vi "Fit Model to Plot Wrapper.vi"(0 "Fit Plot Info":T1, 11 "error in (no error)":errorcluster) -> (1 "Fitted Plot":cluster{"X Array":dbl[], "Y Array":dbl[]}, 2 "Graph Name":string, 3 "Plot Name":string, 4 "Best Fit":dbl[](array[numeric]), 6 "Fit Parameter Names":string[](array[string]), 8 "Additional Parameters":variant, 10 "Fit Parameter Values":dbl[](array[numeric]), 14 "Fit Result String":string, 15 "error out":errorcluster)   [LabVIEW 2021, in "Fits.lvlib"]
uses:
  Fits.lvlib
  Fit Plot Request Information.ctl
  <vilib>/Utility/miscctls.llb/LVPointDoubleTypeDef.ctl
  Fit Models.ctl
  Fit Settings.ctl
  Nonlinear Fit Method.ctl
  IRF(X)PSED/Fit Weights Type v2.ctl
  Ramp Type.ctl
  Residual Type.ctl
  Non-linear Fitting Algorithm.ctl
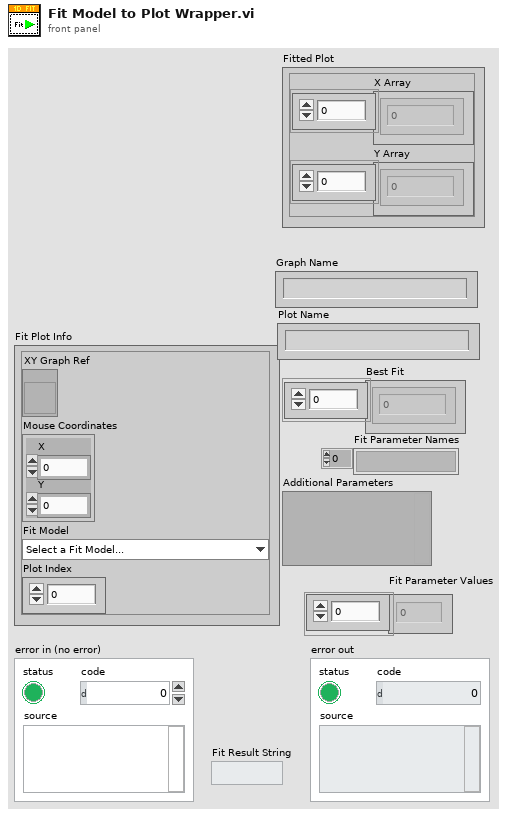
[diagram p1: front panel]
types:
  T1 = typedef "Fits.lvlib/Fit Plot Request Information.ctl" = cluster{"XY Graph Ref":refnum<vi>, "Mouse Coordinates":T2, "Fit Model":T3, "Plot Index":i32}
  T2 = typedef "LVPointDoubleTypeDef.ctl" = cluster{"X":dbl, "Y":dbl}
  T3 = typedef "Fits.lvlib/Fit Models.ctl" = enum16{"Select a Fit Model...", "           Single Peak", "Gaussian", "Asymmetric Gaussian", "Lorentzian", "Asymmetric Lorentzian", "Gaussian/Lorentzian", "Lorentzian/Gaussian", "           Double Peak", "Two Gaussians", "Two Asymmetric Gaussians", "Two H-Connected Gaussians", "Two T-Connected Gaussians", "Two H-Connected Asymmetric Gaussians", "Two T-Connected Asymmetric Gaussians", "           Triple Peak", "Three Gaussians", "Three Asymmetric Gaussians", "              Decays", "1-Exponential", "IRF*PSED", "2-Exponentials", "            Power Law", "Power Law", "Power Law with Offset", "               ACF", "2D Gaussian ACF", "2D Gaussian + Blinking ACF", "2D Gaussian + Flow ACF", "3D Gaussian ACF", "3D Gaussian + Blinking ACF", "             Multiplot", "2D Gaussian ACF & 2D Gaussian + Flow ACF"}
  T4 = typedef "Fits.lvlib/D-Only Fixed Parameters.ctl" = cluster{"Fix D-only Peak Location":bool, "Peak Location":dbl, "Fix D-only Peak FWHM":bool, "Peak FWHM":dbl}
  T5 = typedef "Fits.lvlib/Fit Settings.ctl" = cluster{"Use Original Plot # Points":bool, "# Fit Plot Points":u32, "Fitting Method":T6, "Weighted Fit":T7, "Show All Fit Components":bool, "Axis Type":T8, "Show Fit Residuals":bool, "Residual Type":T9, "Fitting Algorithm":T10, "Show Confidence Interval":bool, "Confidence Level":dbl}
  T6 = typedef "Fits.lvlib/Nonlinear Fit Method.ctl" = enum16{"Least Square", "Least Absolute Residual", "Bisquare", "MLE"}
  T7 = typedef "Fits.lvlib/Fit Weights Type v2.ctl" = enum16{"Unweighted", "1/Variance (Neyman)", "1/Variance (Pearson)", "Best of All"}
  T8 = typedef "Fits.lvlib/Ramp Type.ctl" = u16
  T9 = typedef "Fits.lvlib/Residual Type.ctl" = enum16{"Standard", "Normalized", "Reduced"}
  T10 = typedef "Fits.lvlib/Non-linear Fitting Algorithm.ctl" = enum16{"Levenberg-Marquardt", "Trust-Region Dogleg"}
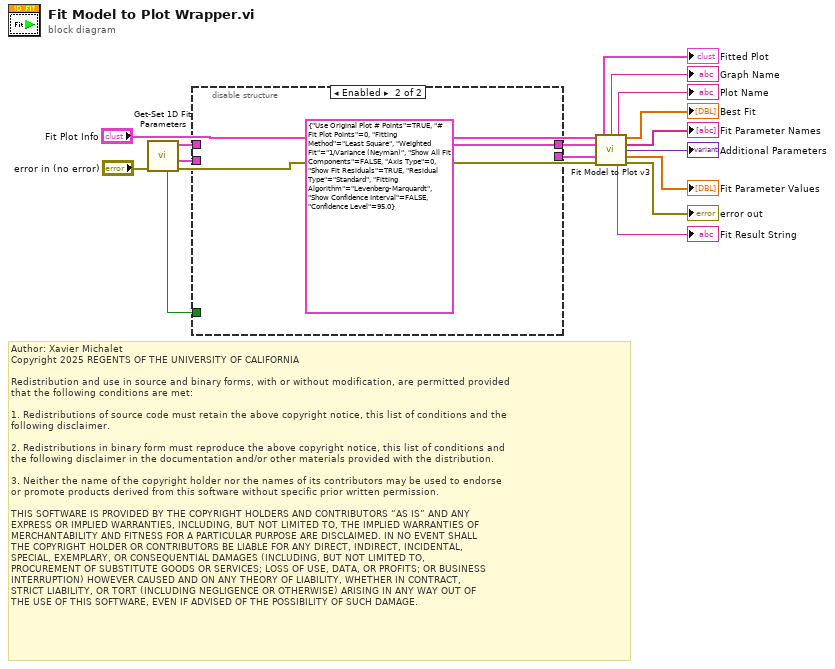
[diagram p0: block diagram]
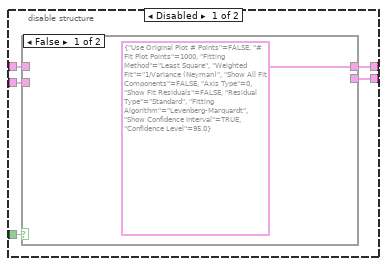
[diagram p2: hidden frame]
diagram:
  # "Author: Xavier Michalet\nCopyright 2025 REGENTS OF THE UNIVERSITY OF CALIFORNIA\n\nRedistribution and use in source and binary forms, with or without modification, are permitted provided\nthat the following conditions are met:\n\n1. Redistributions of source code must retain the above copyright notice, this list of conditions and the\nfollowing disclaimer.\n\n2. Redistributions in binary form must reproduce the above copyright notice, this list of conditions and\nthe following disclaimer in the documentation and/or other materials provided with the distribution.\n\n3. Neither the name of the copyright holder nor the names of its contributors may be used to endorse \nor promote products derived from this software without specific prior written permission.\n\nTHIS SOFTWARE IS PROVIDED BY THE COPYRIGHT HOLDERS AND CONTRIBUTORS “AS IS” AND ANY \nEXPRESS OR IMPLIED WARRANTIES, INCLUDING, BUT NOT LIMITED TO, THE IMPLIED WARRANTIES OF\nMERCHANTABILITY AND FITNESS FOR A PARTICULAR PURPOSE ARE DISCLAIMED. IN NO EVENT SHALL\nTHE COPYRIGHT HOLDER OR CONTRIBUTORS BE LIABLE FOR ANY DIRECT, INDIRECT, INCIDENTAL, \nSPECIAL, EXEMPLARY, OR CONSEQUENTIAL DAMAGES (INCLUDING, BUT NOT LIMITED TO, \nPROCUREMENT OF SUBSTITUTE GOODS OR SERVICES; LOSS OF USE, DATA, OR PROFITS; OR BUSINESS\nINTERRUPTION) HOWEVER CAUSED AND ON ANY THEORY OF LIABILITY, WHETHER IN CONTRACT, \nSTRICT LIABILITY, OR TORT (INCLUDING NEGLIGENCE OR OTHERWISE) ARISING IN ANY WAY OUT OF\nTHE USE OF THIS SOFTWARE, EVEN IF ADVISED OF THE POSSIBILITY OF SUCH DAMAGE."
  n1 = call "Get-Set 1D Fit Parameters.vi"("Error In"="error in (no error)") -> ("Error Out"=w12:errorcluster, "Fixed Parameters"=w16:T4, "Fit Settings"=w14:T5, "Initialized?"=w13:bool)  [unwired: 7 in]
  n2 = disable-structure shown="Enabled" {
    disable-tunnel: w16 -> [w22 _]
    disable-tunnel: [w21 _] -> w15
    disable-tunnel: w14 -> [w20 _]
    disable-tunnel: w13 -> [w19 _]
    disable-tunnel: [w18 T5 {"Use Original Plot # Points"=TRUE, "# Fit Plot Points"=0, "Fitting Method"=enum."Least Square", "Weighted Fit"=enum."1/Variance (Neyman)", "Show All Fit Components"=FALSE, "Axis Type"=0, "Show Fit Residuals"=TRUE, "Residual Type"=enum."Standard", "Fitting Algorithm"=enum."Levenberg-Marquardt", "Show Confidence Interval"=FALSE, "Confidence Level"=95.0} ("Fit Settings")] -> w8
    frame Disabled {
      n3 = case shown="False" w19 {
        tunnel: w20 -> [_ w25]
        tunnel: [T5 {"Use Original Plot # Points"=FALSE, "# Fit Plot Points"=1000, "Fitting Method"=enum."Least Square", "Weighted Fit"=enum."1/Variance (Neyman)", "Show All Fit Components"=FALSE, "Axis Type"=0, "Show Fit Residuals"=FALSE, "Residual Type"=enum."Standard", "Fitting Algorithm"=enum."Levenberg-Marquardt", "Show Confidence Interval"=TRUE, "Confidence Level"=95.0} ("Fit Settings") w25] -> w18
        tunnel: [_ w24] -> w21
        tunnel: w22 -> [_ w24]
        frame False {
        }
        frame True {
        }
      }
    }
    frame Enabled {
    }
  }
  n4 = call "Fit Model to Plot v3.vi"("Fit Plot Information"="Fit Plot Info", "Fit Settings"=w8, "Fixed Parameters"=w15, "error in (no error)"=w12) -> ("Fitted Plot"=→"Fitted Plot":cluster{"X Array":dbl[], "Y Array":dbl[]}, "Graph Name"=→"Graph Name":string, "Plot Name"=→"Plot Name":string, "Best Fit"=→"Best Fit":dbl[], "Fit Parameter Names"=→"Fit Parameter Names":string[], "Additional Parameters (out)"=→"Additional Parameters":variant, "Fit Parameter Values"=→"Fit Parameter Values":dbl[], "Fit Result String"=→"Fit Result String":string, "error out"=→"error out":errorcluster)  [unwired: 3 in]
